vi "Stop Core.vi"(10 "final error code":i32, 11 "server in":refnum<class "server.lvclass">) -> (3 "server out":refnum<class "server.lvclass">)   [LabVIEW 2016, in "server.lvlib" / "server.lvclass"]
doc: "(<B>Filename</B>: Actor Framework.lvlib:Actor.lvclass:Stop Core.vi)\n\nDefines what the actor does before it stops. Use the <B>final error code</B> input to determine whether the actor shut down in response to an error.\n\nBy default, this method does nothing. A descendant class may override it to define behavior, such as shutting down any processes the actor initiated in its override of the Actor Core method."
uses:
  server.lvclass
  server.lvclass/server.ctl
  <vilib>/ActorFramework/Actor/Actor.lvclass
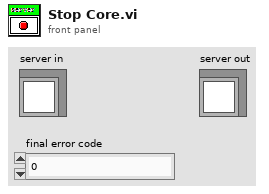
[diagram p1: front panel]
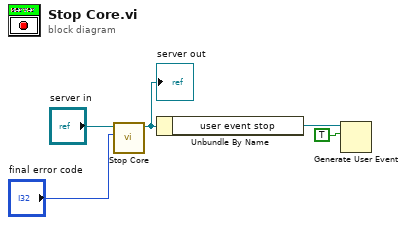
[diagram p0: block diagram]
diagram:
  n1 = call-parent "Stop Core.vi"("final error code"="final error code", "Actor in"="server in") -> ("Actor out"=w3:refnum<class "server.lvclass">)  [unwired: 9 in]
  "server out" <- w3
  n2 = Unbundle By Name(w3) -> ("user event stop"=w2:refnum<user-event>)
  n3 = Generate User Event(user event=w2, event data cluster=TRUE) -> ()  [unwired: 2 in, 2 out]
